vi "Obtain Broadcast Events.vi"(8 "error in (no error)":errorcluster, 10 "Create New? (F)":bool) -> (0 "error out":errorcluster, 2 "Arduino stepper Broadcast Events":T1)   [LabVIEW 2020, in "Arduino stepper.lvlib"]
doc: "This VI Obtains/Creates the Broadcast events that will be used for other modules to register to receive messages from the module that owns this VI.\n\n<b>NOTE</b>: The contents of this VI are automatically generated and modified by the <b>Tools > Delacor > DQMH</b> utilities. Consider using those utilities instead of making your own modifications to this VI.\n_____\nBased on DQMH Project Template 6.1.0.94."
uses:
  Arduino stepper.lvlib
  Broadcast Events--cluster.ctl
  Did Init Argument--cluster.ctl
  Status Updated Argument--cluster.ctl
  Error Reported Argument--cluster.ctl
  Stop Argument--cluster.ctl
  Get Module Execution Status Argument--cluster.ctl
  Device connected Argument--cluster.ctl
  Data available Argument--cluster.ctl
  Info ready Argument--cluster.ctl
  Connection failed Argument--cluster.ctl
  Device disconected Argument--cluster.ctl
  End-position reached Argument--cluster.ctl
  End-stop reached Argument--cluster.ctl
panel:
  # "NOTE: The contents of this VI are automatically generated and modified by the Tools > Delacor > DQMH utilities. Consider using those utilities instead of making your own modifications to this VI."
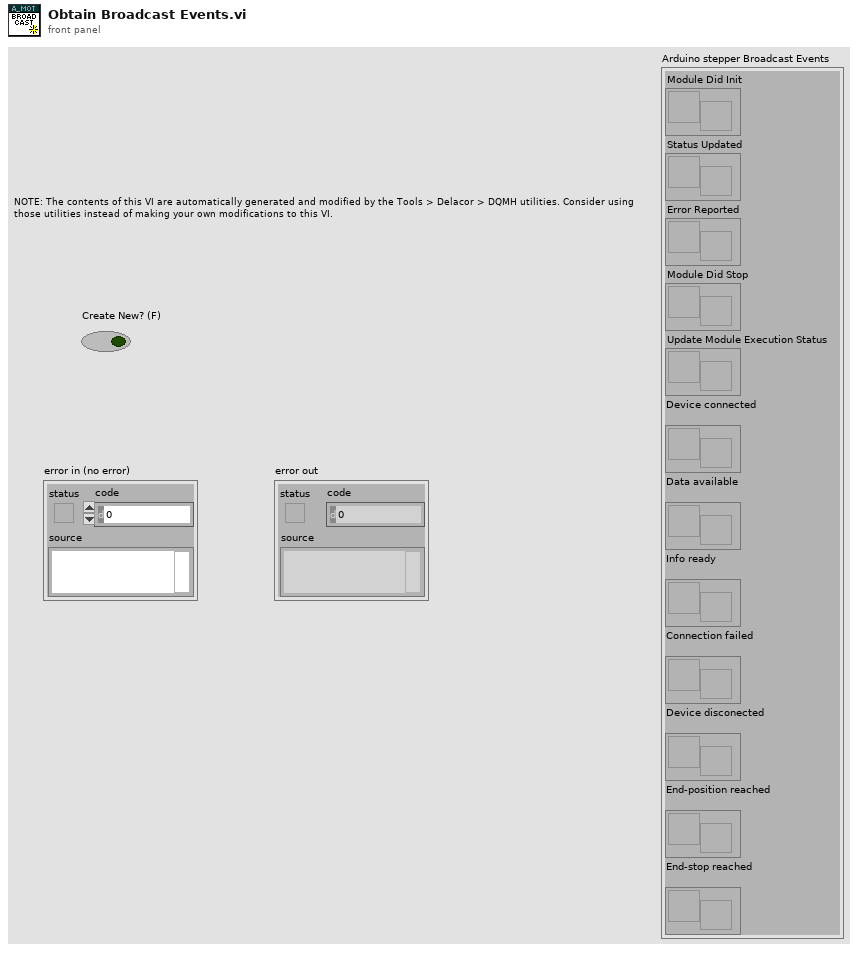
[diagram p1: front panel]
types:
  T1 = typedef "Arduino stepper.lvlib/Broadcast Events--cluster.ctl" = cluster{"Module Did Init":refnum<user-event>, "Status Updated":refnum<user-event>, "Error Reported":refnum<user-event>, "Module Did Stop":refnum<user-event>, "Update Module Execution Status":refnum<user-event>, "Device connected":refnum<user-event>, "Data available":refnum<user-event>, "Info ready":refnum<user-event>, "Connection failed":refnum<user-event>, "Device disconected":refnum<user-event>, "End-position reached":refnum<user-event>, "End-stop reached":refnum<user-event>}
  T2 = typedef "Arduino stepper.lvlib/End-stop reached Argument--cluster.ctl" = cluster{"Module ID":i32, "End-stops":cluster{"ES1":bool, "ES2":bool}}
  T3 = typedef "Arduino stepper.lvlib/End-position reached Argument--cluster.ctl" = cluster{"Module ID":i32, "Boolean":bool}
  T4 = typedef "Arduino stepper.lvlib/Device disconected Argument--cluster.ctl" = cluster{"Module ID":i32, "Connected?":bool}
  T5 = typedef "Arduino stepper.lvlib/Connection failed Argument--cluster.ctl" = cluster{"Module ID":i32, "Connected?":bool, "String":string}
  T6 = typedef "Arduino stepper.lvlib/Info ready Argument--cluster.ctl" = cluster{"Module ID":i32, "Position":i32, "End-stops":cluster{"ES1":bool, "ES2":bool}}
  T7 = typedef "Arduino stepper.lvlib/Data available Argument--cluster.ctl" = cluster{"Module ID":i32, "Data":string}
  T8 = typedef "Arduino stepper.lvlib/Device connected Argument--cluster.ctl" = cluster{"Module ID":i32, "Connected?":bool, "String":string}
  T9 = typedef "Arduino stepper.lvlib/Get Module Execution Status Argument--cluster.ctl" = cluster{"Module ID":i32, "Running?":bool}
  T10 = typedef "Arduino stepper.lvlib/Stop Argument--cluster.ctl" = cluster{"Module ID":i32, "Origin":string, "Exit via Stop Module Req?":bool, "Wait for Module to stop?":bool}
  T11 = typedef "Arduino stepper.lvlib/Error Reported Argument--cluster.ctl" = cluster{"Error":errorcluster, "Additional Information":string, "Module ID":i32, "Module Name":string}
  T12 = typedef "Arduino stepper.lvlib/Status Updated Argument--cluster.ctl" = cluster{"Status":string, "Module ID":i32}
  T13 = typedef "Arduino stepper.lvlib/Did Init Argument--cluster.ctl" = cluster{"Init?":bool, "Info":string, "Module ID":i32}
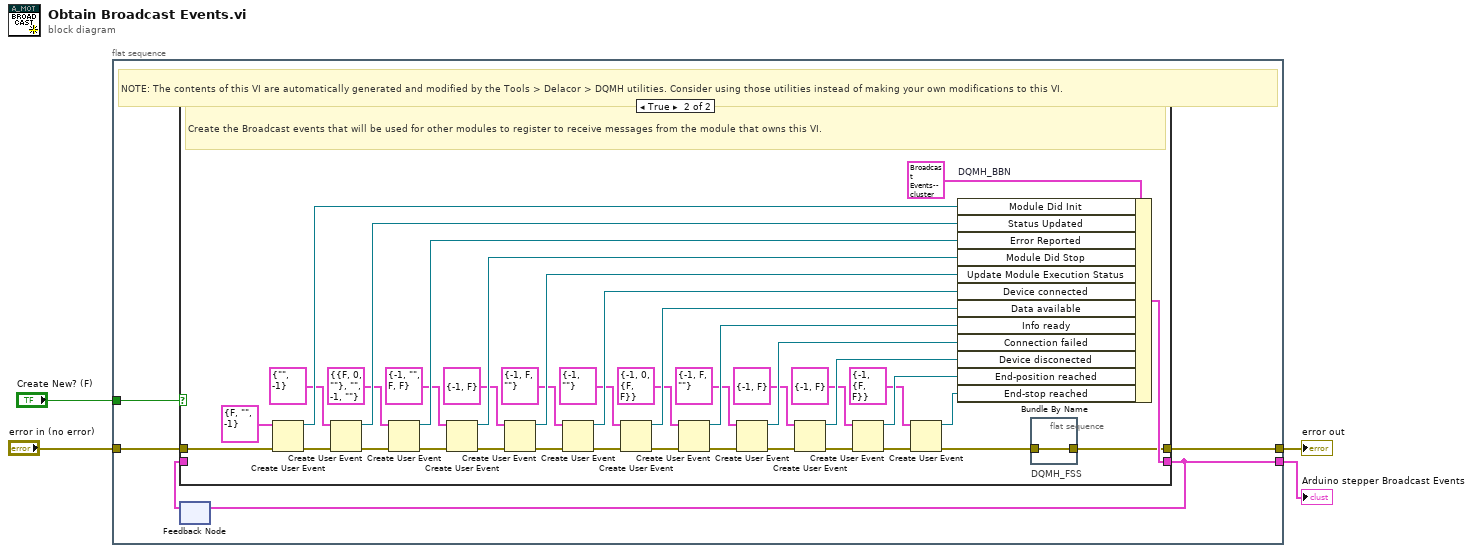
[diagram p0: block diagram]
diagram:
  n1 = flat-sequence {
    tunnel: [w9] -> w4
    tunnel: "error in (no error)" -> [w8]
    tunnel: [w6] -> w2
    tunnel: "Create New? (F)" -> [w5]
    frame #0 {
      # "NOTE: The contents of this VI are automatically generated and modified by the Tools > Delacor > DQMH utilities. Consider using those utilities instead of making your own modifications to this VI."
      n2 = feedback #1() -> (w7:T1)  [unwired: 1 in]
      n3 = case shown="True" w5 {
        tunnel: [w10 w36] -> w9
        tunnel: w8 -> [w10 w51]
        tunnel: [w11 w48] -> w6
        tunnel: w7 -> [w11 _]
        frame False {
          # "Obtain the Broadcast events that were created in a previous call to this VI."
        }
        frame True {
          # "Create the Broadcast events that will be used for other modules to register to receive messages from the module that owns this VI."
          n4 = Create User Event(user event datatype=T13 {"Init?"=FALSE, "Info"="", "Module ID"=-1} ("Did Init Argument"), error in=w51) -> (user event=w49:refnum<user-event>, error out=w46:errorcluster)
          n5 = Create User Event(user event datatype=T12 {"Status"="", "Module ID"=-1} ("Status Updated Argument"), error in=w46) -> (user event=w43:refnum<user-event>, error out=w45:errorcluster)
          n6 = Create User Event(user event datatype=T11 {"Error"={"status"=FALSE, "code"=0, "source"=""}, "Additional Information"="", "Module ID"=-1, "Module Name"=""} ("Error Reported Argument"), error in=w45) -> (user event=w40:refnum<user-event>, error out=w42:errorcluster)
          n7 = Create User Event(user event datatype=T10 {"Module ID"=-1, "Origin"="", "Exit via Stop Module Req?"=FALSE, "Wait for Module to stop?"=FALSE} ("Stop Argument"), error in=w42) -> (user event=w38:refnum<user-event>, error out=w37:errorcluster)
          n8 = Create User Event(user event datatype=T9 {"Module ID"=-1, "Running?"=FALSE} ("Get Module Execution Status Argument"), error in=w37) -> (user event=w34:refnum<user-event>, error out=w35:errorcluster)
          n9 = Create User Event(user event datatype=T8 {"Module ID"=-1, "Connected?"=FALSE, "String"=""} ("Device connected Argument"), error in=w35) -> (user event=w31:refnum<user-event>, error out=w32:errorcluster)
          n10 = Create User Event(user event datatype=T7 {"Module ID"=-1, "Data"=""} ("Data available Argument"), error in=w32) -> (user event=w28:refnum<user-event>, error out=w29:errorcluster)
          n11 = Create User Event(user event datatype=T6 {"Module ID"=-1, "Position"=0, "End-stops"={"ES1"=FALSE, "ES2"=FALSE}} ("Info ready Argument"), error in=w29) -> (user event=w25:refnum<user-event>, error out=w26:errorcluster)
          n12 = Create User Event(user event datatype=T5 {"Module ID"=-1, "Connected?"=FALSE, "String"=""} ("Connection failed Argument"), error in=w26) -> (user event=w22:refnum<user-event>, error out=w23:errorcluster)
          n13 = Create User Event(user event datatype=T4 {"Module ID"=-1, "Connected?"=FALSE} ("Device disconected Argument"), error in=w23) -> (user event=w19:refnum<user-event>, error out=w20:errorcluster)
          n14 = Create User Event(user event datatype=T3 {"Module ID"=-1, "Boolean"=FALSE} ("End-position reached Argument"), error in=w20) -> (user event=w16:refnum<user-event>, error out=w17:errorcluster)
          n15 = Create User Event(user event datatype=T2 {"Module ID"=-1, "End-stops"={"ES1"=FALSE, "ES2"=FALSE}} ("End-stop reached Argument"), error in=w17) -> (user event=w13:refnum<user-event>, error out=w14:errorcluster)
          n16 = Bundle By Name "DQMH_BBN"(cluster=T1 {"Module Did Init"=refnum, "Status Updated"=refnum, "Error Reported"=refnum, "Module Did Stop"=refnum, "Update Module Execution Status"=refnum, "Device connected"=refnum, "Data available"=refnum, "Info ready"=refnum, "Connection failed"=refnum, "Device disconected"=refnum, "End-position reached"=refnum, "End-stop reached"=refnum} ("output cluster"), "Module Did Init"=w49, "Status Updated"=w43, "Error Reported"=w40, "Module Did Stop"=w38, "Update Module Execution Status"=w34, "Device connected"=w31, "Data available"=w28, "Info ready"=w25, "Connection failed"=w22, "Device disconected"=w19, "End-position reached"=w16, "End-stop reached"=w13) -> (w48:T1)
          n17 = flat-sequence "DQMH_FSS" {
            tunnel: w14 -> [w52]
            tunnel: [w52] -> w36
            frame #0 {
            }
          }
        }
      }
      n18 = feedback-in #1(w6) -> ()
    }
  }
  "Arduino stepper Broadcast Events" <- w2
  "error out" <- w4
